vi "QSM_CreateRef.vi"(8 "error in":errorcluster) -> (0 "error out":errorcluster, 3 "QSM_Reference out":T1)   [LabVIEW 2014, in "GUIUpdateQSM.lvlib"]
doc: "VARIABLE FREQUENCY DRIVE CONTROL 'VFDC' Queued State Machine Shift Register Data:\n\nThe data type for the main shift register in the subsequent queued state machine is defined in large clusters within this VI."
uses:
  GUIUpdateQSM.lvlib
  Controls/QSM_Reference.ctl
  Controls/QSM_DataType.ctl
  Controls/QSM_RunStates.ctl
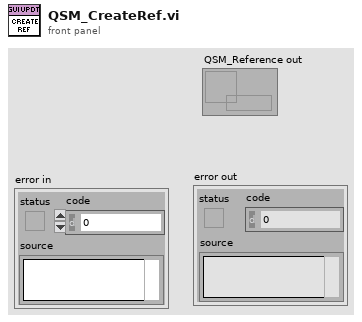
[diagram p1: front panel]
types:
  T1 = typedef "GUIUpdateQSM.lvlib/QSM_Reference.ctl" = refnum<queue>
  T2 = typedef "GUIUpdateQSM.lvlib/QSM_DataType.ctl" = cluster{"QSM_RunStates":T3, "DATA.VARIANT":variant}
  T3 = typedef "GUIUpdateQSM.lvlib/QSM_RunStates.ctl" = enum16{"NULL", "Sect01_Initialize-00_GROUP.ENQUEUE", "Sect01_Initialize-01_SetMainToDefault", "Sect01_Initialize-02_Clear Status Strings", "Sect02_UpdateUI-00_Enable Stop_ Disable Start", "Sect02_UpdateUI-01_Enable Start_Disable Stop", "Sect02_UpdateUI-02_Update Status String", "Sect02_UpdateUI-03_Clear XY-Graph", "Sect03-Open ROI  GUI", "Sect03-Close ROI GUI", "Sect99_EXIT-00_Group.Enqueue", "Sect99_EXIT-01_CloseReferences", "Sect99_EXIT-02_StopQSM"}
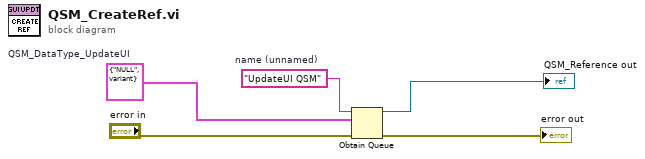
[diagram p0: block diagram]
diagram:
  w2 = T2 {"QSM_RunStates"=enum."NULL", "DATA.VARIANT"=variant}  # QSM_DataType_UpdateUI
  w3 = "UpdateUI QSM"  # name (unnamed)
  n1 = Obtain Queue ("Obtain Queues")(name (unnamed)=w3, element data type=w2, error in (no error)="error in") -> (queue out=→"QSM_Reference out":refnum<queue>, error out=→"error out":errorcluster)  [unwired: 2 in, 1 out]
